vi "test_232_imu_MW-AHRSv1_3d-2.vi"() -> ()   [LabVIEW 2019]
uses:
  <vilib>/Utility/miscctls.llb/LV3DPointTypeDef.ctl
  Ctrl/cmd_imu.ctl
  <vilib>/Instr/_visa.llb/VISA Configure Serial Port (Instr).vi
  <vilib>/picture/3D Picture Control/Object/Create Object (name).vi
  <vilib>/picture/3D Picture Control/Object/Add Object (no reference).vi
  <vilib>/picture/3D Picture Control/Object/Create Object (drawable).vi
  <vilib>/picture/3D Picture Control/NI_3D Picture Control.lvlib
panel:
  out "error out 2":errorcluster
  in  "baud rate":u32=115200 caption="rate"
  in  "Port":refnum<visa-resource-name>="COM24"
  out "r buff":u32(graph)
  in  "w-data":string="ang"
  in  "w":bool
  in  "reset":bool
  out "heading":dbl format="%.1f"
  in  "Stop":bool
  in  "Draw Mode":T1(ring)=enum."Polygons"
  in  "Color":u32(colorbox)=16860
  in  "Half plane?":bool=TRUE
  in  "show axis":bool=TRUE
  in  "Size":dbl=-1.0
  in  "Axis label?":bool=TRUE
  out "3D Picture":refnum<vi>(3d-picture)
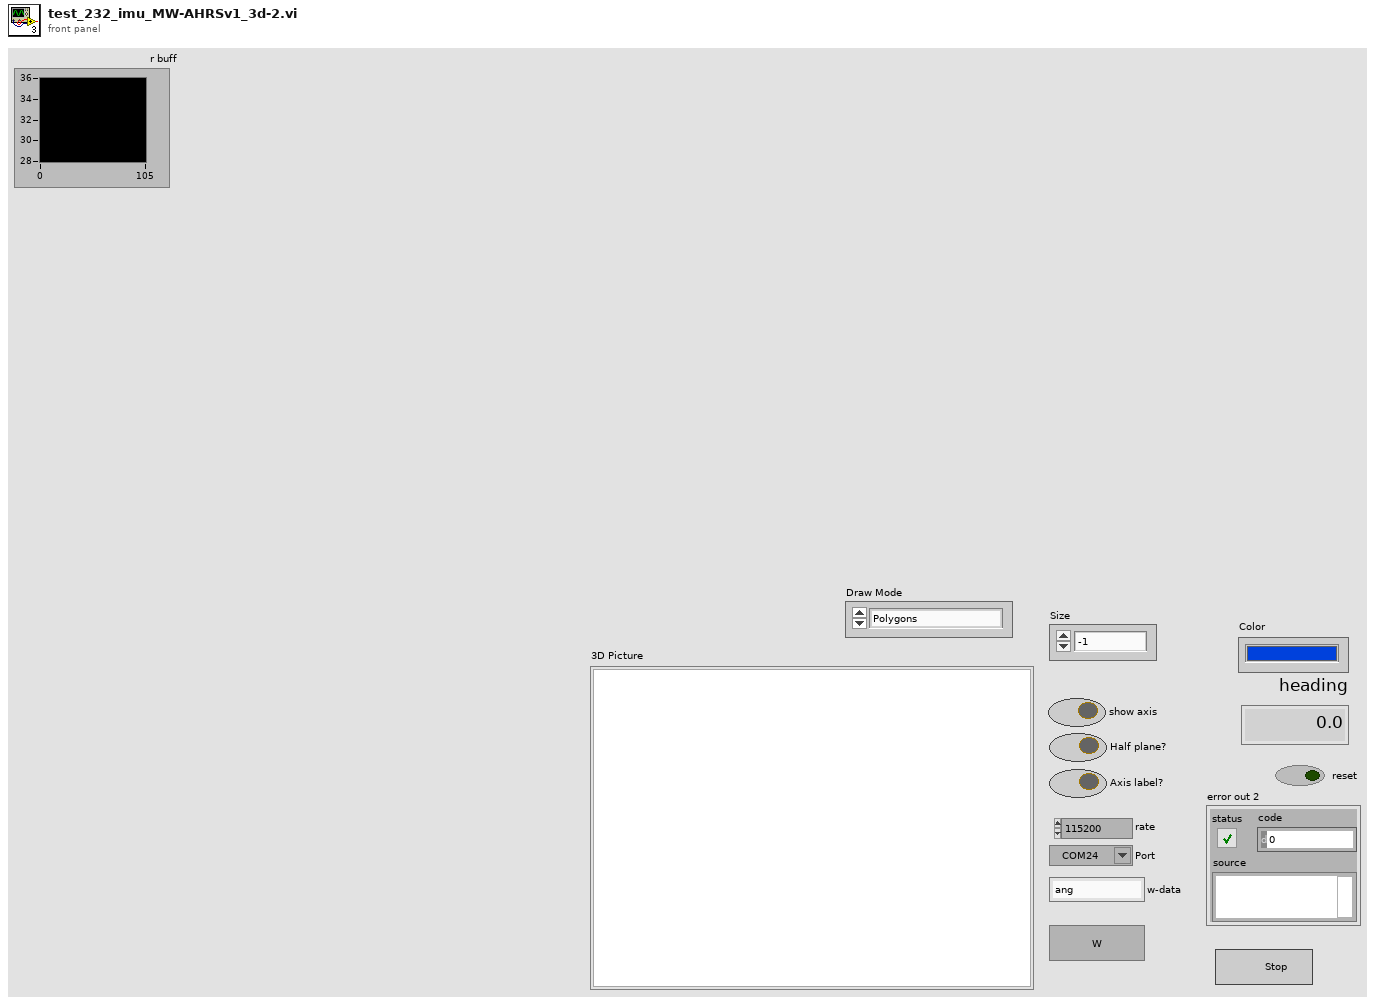
[diagram p1: front panel]
types:
  T1 = enum16{"Inherit Value", "Points", "Wireframe", "Polygons"}
  T2 = typedef "LV3DPointTypeDef.ctl" = cluster{"X":sgl, "Y":sgl, "Z":sgl}
  T3 = typedef "cmd_imu.ctl" = enum16{"ini", "write", "read"}
  T4 = cluster{"angle":dbl[], "acc":dbl[], "mag":dbl[], "gyr":dbl[]}
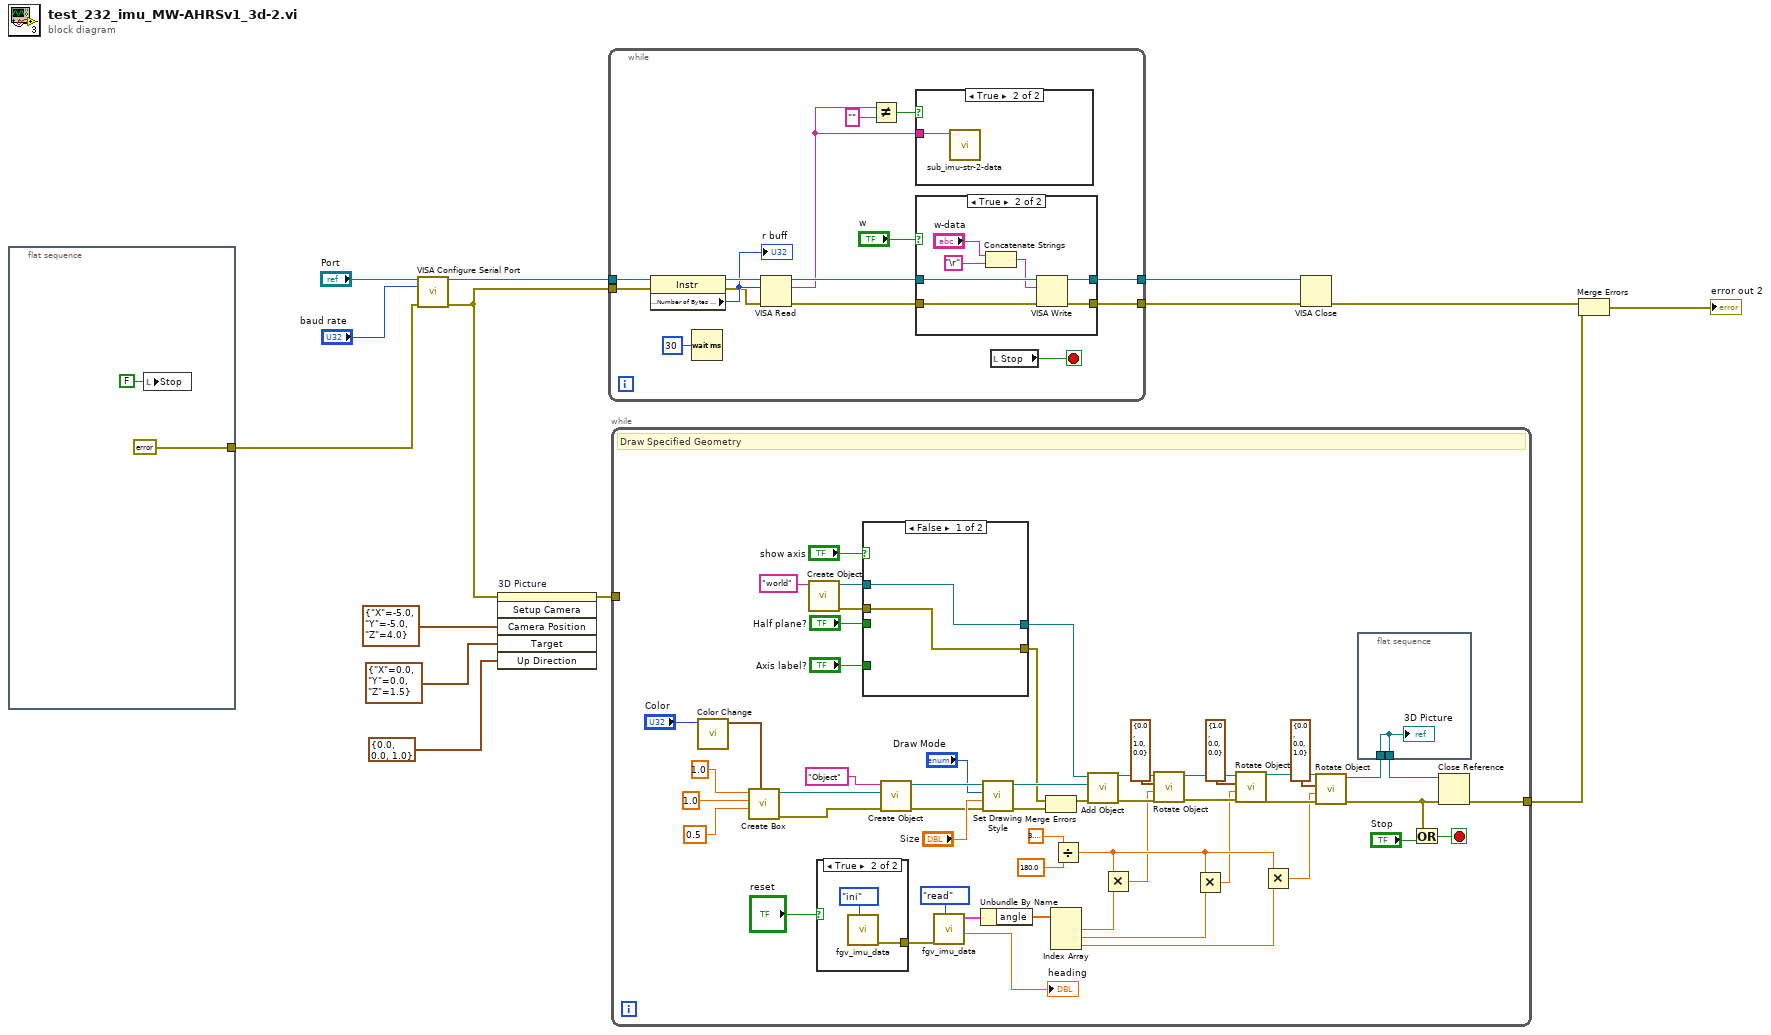
[diagram p0: block diagram]
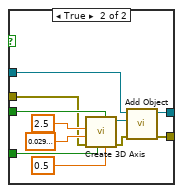
[diagram p5: hidden frame]
diagram:
  n1 = flat-sequence {
    tunnel: [errorcluster {"status"=FALSE, "code"=0, "source"=""} ("error in (no error)")] -> w4
    frame #0 {
      n2 = local write "Stop"(FALSE ("Stop")) -> ()
    }
  }
  n3 = call-poly "VISA Configure Serial Port"("VISA resource name"="Port", "baud rate (9600)"="baud rate", "error in (no error)"=w4) -> ("VISA resource name out"=w6:refnum<visa-resource-name>, "error out"=w5:errorcluster)  [unwired: 11 in]
  n4 = invoke on="3D Picture" class="SceneGraphDisp (strict)" method="Setup Camera"(error in=w5, "Camera Position"=T2 {"X"=-5.0, "Y"=-5.0, "Z"=4.0}, "Target"=T2 {"X"=0.0, "Y"=0.0, "Z"=1.5} ("Camera Position"), "Up Direction"=T2 {"X"=0.0, "Y"=0.0, "Z"=1.0}) -> (error out=w14:errorcluster)  [unwired: 2 in, 5 out]
  n5 = while {
    tunnel: w5 -> [w27]
    tunnel: w6 -> [w26]
    tunnel: [w22] -> w10
    tunnel: [w21] -> w9
    stop <- w17 stop-if-true
    n6 = property class="Instr"(reference=w26, error in=w27) -> (reference out=w31:refnum<visa-resource-name>, error out=w28:errorcluster, "Serial Settings:Number of Bytes at Serial Port"=w29:u32)
    "r buff" <- w29
    n7 = Wait (ms)(milliseconds to wait=u32 30 ("대기 시간 (ms)")) -> ()  [unwired: 1 out]
    n8 = VISA Read(VISA resource name=w31, byte count=w29, error in (no error)=w28) -> (VISA resource name out=w23:refnum<visa-resource-name>, read buffer=w18:string, error out=w24:errorcluster)  [unwired: 1 out]
    n9 = Not Equal?(x=w18, y="") -> (x != y?=w20:bool)
    n10 = case shown="True" w20 {
      tunnel: w18 -> [_ w32]
      frame False {
      }
      frame True {
        n11 = call "sub_imu-str-2-data.vi"("read buffer"=w32) -> ()  [unwired: 9 in, 2 out]
      }
    }
    n12 = case shown="True" "w" {
      tunnel: w23 -> [w34 w41]
      tunnel: [w34 w40] -> w22
      tunnel: w24 -> [w33 w39]
      tunnel: [w33 w38] -> w21
      frame False {
      }
      frame True {
        n13 = Concatenate Strings("w-data", "\r") -> (w35:string)
        n14 = VISA Write(VISA resource name=w41, write buffer=w35, error in (no error)=w39) -> (VISA resource name out=w40:refnum<visa-resource-name>, error out=w38:errorcluster)  [unwired: 1 out]
      }
    }
    n15 = local read "Stop"() -> (w17:bool)
  }
  n16 = while {
    tunnel: w14 -> [_]
    tunnel: [w44] -> w2
    stop <- w85 stop-if-true
    # "Draw Specified Geometry"
    n17 = call <vilib>:"Color Change.vi"("Color"="Color") -> ("RGBA"=w91:cluster{"R":sgl, "G":sgl, "B":sgl, "A":sgl})  [unwired: 10 in]
    n18 = call <vilib>:"Create Box.vi"("Color"=w91, "Length Z"=sgl 0.5, "Length Y"=sgl 1.0, "Length X"=sgl 1.0) -> ("error out"=w86:errorcluster, "New Box Refnum"=w93:refnum<vi>)  [unwired: 6 in]
    n19 = call-poly <vilib>:"Create Object.vi"("Name"="world") -> ("error out"=w73:errorcluster, "Scene:New Object"=w74:refnum<vi>)  [unwired: 9 in]
    n20 = case shown="True" "reset" {
      tunnel: [_ w95] -> w52
      frame False {
      }
      frame True {
        n21 = call "fgv_imu_data.vi"("cmd"=cmd_imu."ini") -> ("error out"=w95:errorcluster)  [unwired: 7 in, 3 out]
      }
    }
    n22 = case shown="False" "show axis" {
      tunnel: [w99 w103] -> w89
      tunnel: "Half plane?" -> [_ w108]
      tunnel: [w98 w100] -> w78
      tunnel: "Axis label?" -> [_ w107]
      tunnel: w74 -> [w99 w105]
      tunnel: w73 -> [w98 w102]
      frame False {
        # "Pass an empty model when displaying no axis."
      }
      frame True {
        # "Add a 3D axis."
        n23 = call <vilib>:"Create 3D Axis.vi"("Character Size"=sgl 0.5, "Half plane?"=w108, "Axis label?"=w107, "error in (no error)"=w102, "Radius"=sgl 0.03, "Length"=sgl 2.5 ("Height")) -> ("error out"=w101:errorcluster, "New Object Refnum"=w104:refnum<vi>)  [unwired: 4 in]
        n24 = call-poly <vilib>:"Add Object.vi"("error in (no error)"=w101, "New Object In"=w104, "Scene Object In"=w105) -> ("error out"=w100:errorcluster, "Scene Object Out"=w103:refnum<vi>)  [unwired: 7 in]
      }
    }
    n25 = call-poly <vilib>:"Create Object.vi"("error in (no error)"=w86, "Geometry"=w93, "Name"="Object") -> ("error out"=w76:errorcluster, "Scene:New Object"=w84:refnum<vi>)  [unwired: 7 in]
    n26 = call "fgv_imu_data.vi"("cmd"=cmd_imu."read", "error in"=w52) -> ("heading"=→"heading":dbl, "IMD data out"=w56:T4)  [unwired: 6 in, 2 out]
    n27 = Unbundle By Name(w56) -> ("angle"=w55:dbl[])
    n28 = call <vilib>:"Set Drawing Style.vi"("error in (no error)"=w76, "Size"="Size", "Mode"="Draw Mode", "Scene Object In"=w84) -> ("error out"=w80:errorcluster, "Scene Object Out"=w83:refnum<vi>)  [unwired: 6 in]
    n29 = Merge Errors(w78, w80) -> (w79:errorcluster)
    n30 = Index Array(array=w55) -> (element #1=w48:dbl, element #2=w47:dbl, element #3=w46:dbl)  [unwired: 3 in]
    n31 = Divide(x=3.141592653589793, y=180.0) -> (x/y=w49:dbl)
    n32 = call-poly <vilib>:"Add Object.vi"("error in (no error)"=w79, "New Object In"=w83, "Scene Object In"=w89) -> ("error out"=w59:errorcluster, "Scene Object Out"=w60:refnum<vi>)  [unwired: 7 in]
    n33 = Multiply(x=w49, y=w48) -> (x*y=w45:dbl)
    n34 = call <vilib>:"Rotate Object.vi"("error in (no error)"=w59, "Angle"=w45, "Axis"=cluster{"X":sgl, "Y":sgl, "Z":sgl} {"X"=0.0, "Y"=1.0, "Z"=0.0}, "Scene.Object In"=w60) -> ("error out"=w67:errorcluster, "Scene.Object Out"=w68:refnum<vi>)  [unwired: 6 in]
    n35 = Multiply(x=w49, y=w47) -> (x*y=w42:dbl)
    n36 = call <vilib>:"Rotate Object.vi"("error in (no error)"=w67, "Angle"=w42, "Axis"=cluster{"X":sgl, "Y":sgl, "Z":sgl} {"X"=1.0, "Y"=0.0, "Z"=0.0}, "Scene.Object In"=w68) -> ("error out"=w64:errorcluster, "Scene.Object Out"=w65:refnum<vi>)  [unwired: 6 in]
    n37 = Multiply(x=w49, y=w46) -> (x*y=w43:dbl)
    n38 = call <vilib>:"Rotate Object.vi"("error in (no error)"=w64, "Angle"=w43, "Axis"=cluster{"X":sgl, "Y":sgl, "Z":sgl} {"X"=0.0, "Y"=0.0, "Z"=1.0}, "Scene.Object In"=w65) -> ("error out"=w58:errorcluster, "Scene.Object Out"=w61:refnum<vi>)  [unwired: 6 in]
    n39 = flat-sequence {
      tunnel: w61 -> [w97]
      tunnel: [w97] -> w72
      frame #0 {
        "3D Picture" <- w97
      }
    }
    n40 = Or(x=w58, y="Stop") -> (x .or. y?=w85:bool)
    n41 = Close Reference(reference=w72, error in (no error)=w58) -> (error out=w44:errorcluster)
  }
  n42 = VISA Close(VISA resource name=w10, error in (no error)=w9) -> (error out=w3:errorcluster)
  n43 = Merge Errors(w3, w2) -> (→"error out 2":errorcluster)
